vi "Set Log File Segmenting by Size.vi"(8 "error in":errorcluster, 9 "file size (MB)":u32=10, 10 "segment into multiple files":bool=TRUE, 11 "log file in":T1 format="%.0x") -> (0 "error out":errorcluster, 3 "log file out":T1 format="%.0x")   [LabVIEW 2027, in "Embedded Data Logger Scripting.lvlib"]
uses:
  Embedded Data Logger Scripting.lvlib
  <vilib>/NI VeriStand/Custom Device API/Custom Device Item Ref.ctl
  Shared/Segment Files By.ctl
  Shared/Constants.vi
  <vilib>/NI VeriStand/Custom Device API/Set Item Property (U32).vi
  <vilib>/NI VeriStand/Custom Device API/Set Item Property (Boolean).vi
  <vilib>/NI VeriStand/Custom Device API/Set Item Property (U16).vi
  Shared/Embedded Data Logger Shared.lvlib
  <vilib>/NI VeriStand/Custom Device API/Custom Device API.lvlib
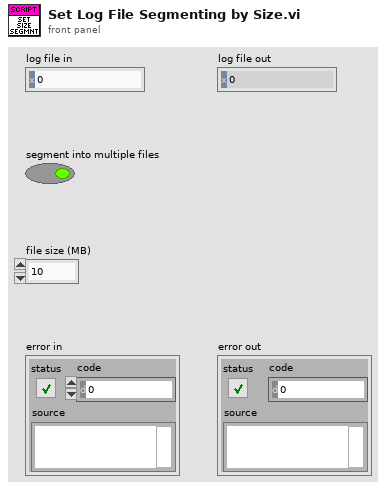
[diagram p1: front panel]
types:
  T1 = typedef "Custom Device API.lvlib/Custom Device Item Ref.ctl" = u64
  T2 = typedef "Embedded Data Logger Shared.lvlib/Segment Files By.ctl" = enum16{"Time", "Size"}
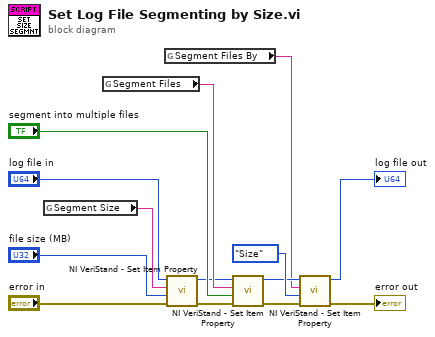
[diagram p0: block diagram]
diagram:
  n1 = global read "Constants.vi" "Segment Size"() -> (w5:string)
  n2 = global read "Constants.vi" "Segment Files"() -> (w8:string)
  n3 = global read "Constants.vi" "Segment Files By"() -> (w1:string)
  n4 = call-poly <vilib>:"NI VeriStand - Set Item Property.vi"("error in (no error)"="error in", "Value"="file size (MB)", "Property Name"=w5, "Item Ref in"="log file in") -> ("error out"=w6:errorcluster, "Item Ref out"=w7:T1)  [unwired: 5 in, 1 out]
  n5 = call-poly <vilib>:"NI VeriStand - Set Item Property.vi"("error in (no error)"=w6, "Value"="segment into multiple files", "Property Name"=w8, "Item Ref in"=w7) -> ("error out"=w10:errorcluster, "Item Ref out"=w11:T1)  [unwired: 5 in, 1 out]
  n6 = call-poly <vilib>:"NI VeriStand - Set Item Property.vi"("error in (no error)"=w10, "Value"=Segment_Files_By."Size" ("Segment Files By"), "Property Name"=w1, "Item Ref in"=w11) -> ("error out"=→"error out":errorcluster, "Item Ref out"=→"log file out":T1)  [unwired: 5 in, 1 out]
